vi "ParticleSwarmCore.vi"(4 "Stop notifier":refnum<notifier>, 5 "Fitness Function Data":variant, 6 "Parameters":T1={"Swarm size"=100, "Generations no."=500, "Cognitive coeff a1"=6.0, "Social coeff a2"=0.85, "Min inertia weight"=0.0, "Max inertia weight "=0.9, "Fmax"=0} {"Generations no." min=1; "Swarm size" min=1}, 7 "Fitness Function":T2, 8 "Population notifier":refnum<notifier>, 9 "Solution Progress notifier":refnum<notifier>, 10 "Satysfing fitness":dbl=inf, 11 "Phenotype size":i32) -> (0 "Generation":i32, 1 "fitness":dbl, 3 "Solution":i32[](array[numeric]))   [LabVIEW 2016, in "Optimal Frequency Bands Search.lvlib" / "ParticleSwarm.lvlib"]
doc: "Процедура, реализующая алгоритм роя частиц."
uses:
  ParticleSwarm.lvlib
  tFitness Function.ctl
  PSO_tParameters.ctl
  PSO_tPopulation.ctl
  PSO_tSolution progress.ctl
panel:
  # "This VI is a part of BCI Design library, http://www.ru-bci.org \nCopyright © 2020, Sotnikov Peter, All rights reserved. License: GNU GPLv3"
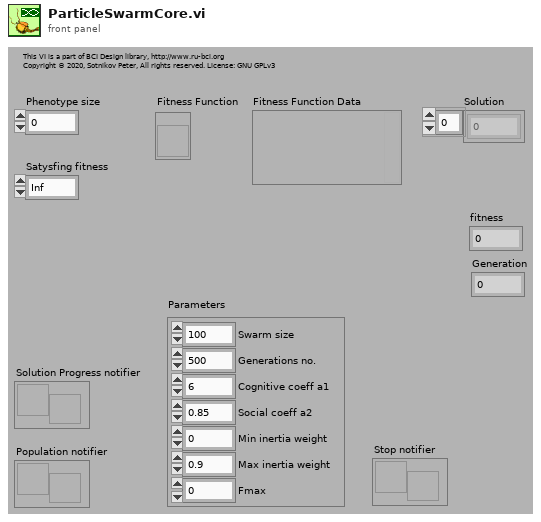
[diagram p1: front panel]
types:
  T1 = typedef "Optimal Frequency Bands Search.lvlib/ParticleSwarm.lvlib/PSO_tParameters.ctl" = cluster{"Swarm size":i32, "Generations no.":i32, "Cognitive coeff a1":dbl, "Social coeff a2":dbl, "Min inertia weight":dbl, "Max inertia weight ":dbl, "Fmax":i32}
  T2 = typedef "Optimal Frequency Bands Search.lvlib/ParticleSwarm.lvlib/tFitness Function.ctl" = refnum<vi>
  T3 = typedef "Optimal Frequency Bands Search.lvlib/ParticleSwarm.lvlib/PSO_tSolution progress.ctl" = cluster{"Solution":i32[], "Fitness":dbl, "Inertia":dbl, "Generation":i32}
  T4 = typedef "Optimal Frequency Bands Search.lvlib/ParticleSwarm.lvlib/PSO_tPopulation.ctl" = cluster{"Particle Coordinates":i32[][], "Fitnesses":dbl[], "Sorted indices":i32[], "Pbest Fitnesses":dbl[], "Pbest Particle Coordinates":i32[][], "Previous Velocity":dbl[][]}
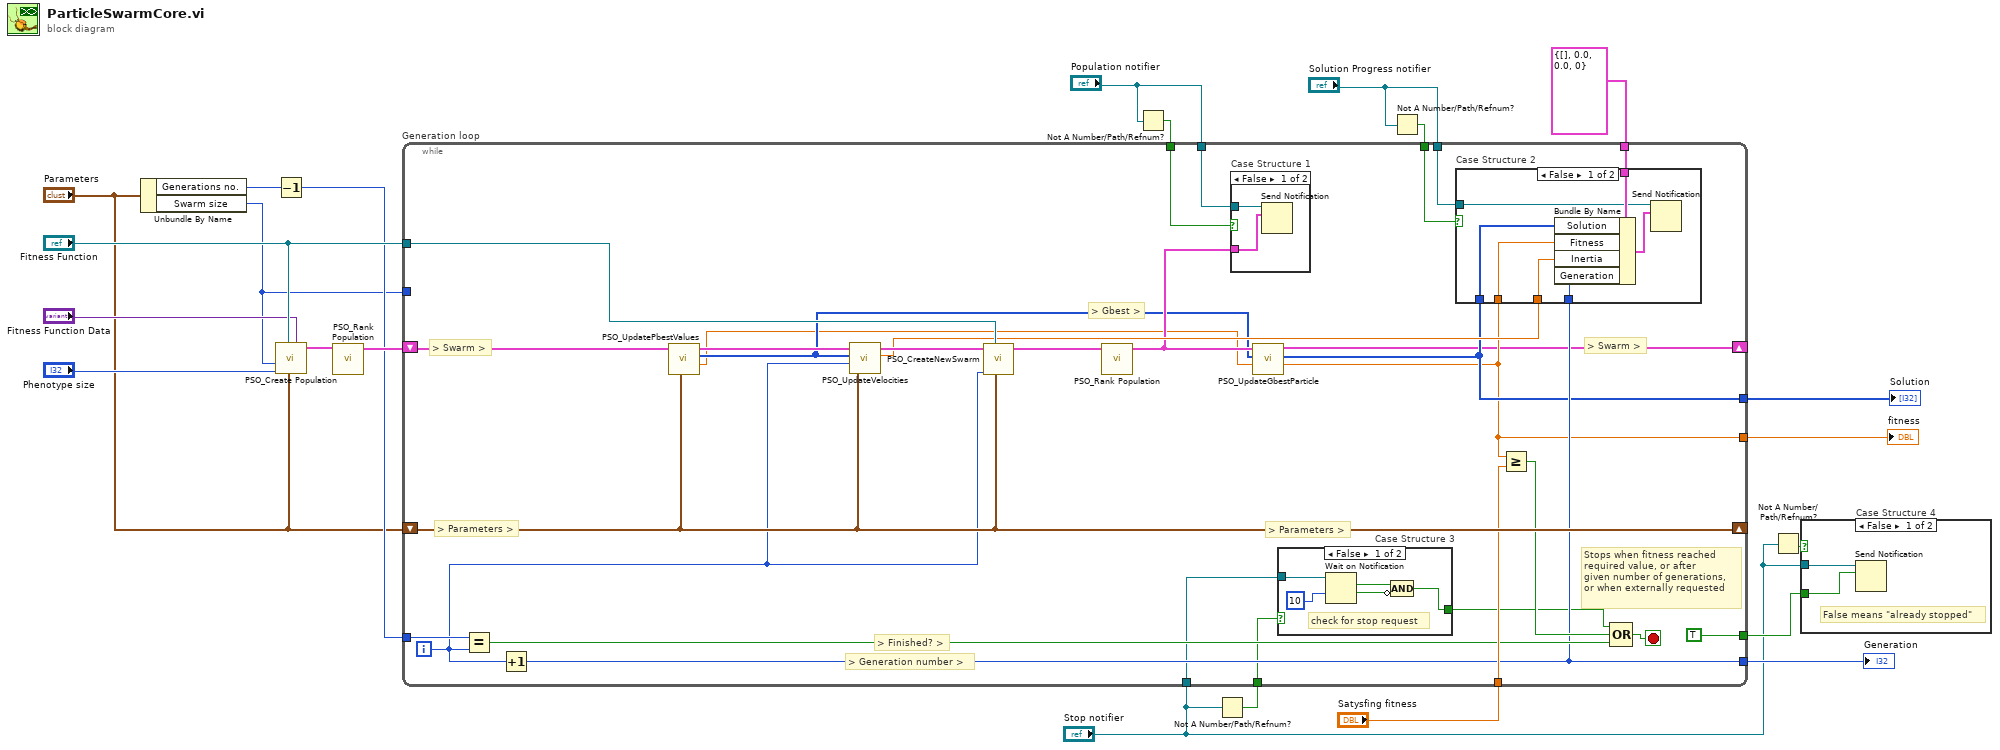
[diagram p0: block diagram]
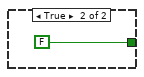
[diagram p3: hidden frame]
diagram:
  n1 = Unbundle By Name("Parameters") -> ("Generations no."=w17:i32, "Swarm size"=w4:i32)
  n2 = Decrement(x=w17) -> (x-1=w16:i32)
  n3 = call "PSO_Create Population.vi"("Function Data"="Fitness Function Data", "Parameters"="Parameters", "Fitness Function"="Fitness Function", "Phenotype size"="Phenotype size", "Population size"=w4) -> ("Population out"=w21:T4)  [unwired: 6 in]
  n4 = call "PSO_Rank Population.vi"("Population in"=w21) -> ("Population out"=w20:T4)  [unwired: 10 in]
  n5 = Not A Number/Path/Refnum?(number/path/refnum="Population notifier") -> (NaN/Path/Refnum?=w9:bool)
  n6 = Not A Number/Path/Refnum?(number/path/refnum="Stop notifier") -> (NaN/Path/Refnum?=w5:bool)
  n7 = Not A Number/Path/Refnum?(number/path/refnum="Solution Progress notifier") -> (NaN/Path/Refnum?=w7:bool)
  n8 = while "Generation loop" {
    tunnel: w4 -> [_]
    shift-right: [w24] -> _
    shift-left: w20 -> [w50]
    shift-right: [w51] -> _
    shift-left: "Parameters" -> [w51]
    tunnel: "Fitness Function" -> [w49]
    tunnel: w16 -> [w48]
    tunnel: "Satysfing fitness" -> [w47]
    tunnel: "Population notifier" -> [w38]
    tunnel: T3 {"Solution"=[], "Fitness"=0.0, "Inertia"=0.0, "Generation"=0} ("Solution progress") -> [w43]
    tunnel: [w42] -> w14
    tunnel: "Solution Progress notifier" -> [w37]
    tunnel: "Stop notifier" -> [w39]
    tunnel: [TRUE] -> w11
    tunnel: w9 -> [w36]
    tunnel: w7 -> [w35]
    tunnel: w5 -> [w34]
    tunnel: [w26] -> w3
    tunnel: [w25] -> w2
    i -> [w23]
    stop <- w46 stop-if-true
    # "> Gbest >"
    # "> Finished? >"
    # "> Generation number >"
    # "Stops when fitness reached\nrequired value, or after\ngiven number of generations,\nor when externally requested"
    # "> Parameters >"
    # "> Swarm >"
    # "> Parameters >"
    # "> Swarm >"
    n9 = Equal?(x=w48, y=w23) -> (x = y?=w45:bool)
    n10 = Increment(x=w23) -> (x+1=w42:i32)
    n11 = call "PSO_UpdatePbestValues.vi"("Parameters"=w51, "Population in"=w50) -> ("GBest Fitness"=w27:dbl, "Gbest Particle"=w28:i32[], "Population out"=w33:T4)  [unwired: 7 in]
    n12 = call "PSO_UpdateVelocities.vi"("Parameters in"=w51, "Generation"=w23, "Gbest Particle"=w28, "Population"=w33) -> ("Inertia Weight"=w30:dbl, "Population out"=w32:T4)  [unwired: 6 in]
    n13 = call "PSO_CreateNewSwarm.vi"("Parameters"=w51, "Fitness Function"=w49, "Generation"=w23, "Population in"=w32) -> ("Population out"=w31:T4)  [unwired: 7 in]
    n14 = call "PSO_Rank Population.vi"("Population in"=w31) -> ("Population out"=w29:T4)  [unwired: 10 in]
    n15 = case "Case Structure 1" shown="False" w36 {
      tunnel: w38 -> [w66 _]
      tunnel: w29 -> [w65 _]
      frame False {
        n16 = Send Notification(notification=w65, notifier=w66) -> ()  [unwired: 1 in, 2 out]
      }
      frame True {
      }
    }
    n17 = call "PSO_UpdateGbestParticle.vi"("Gbest Fitness"=w27, "Gbest Particle"=w28, "Population in"=w29) -> ("Fitness"=w25:dbl, "Solution"=w26:i32[], "Population out"=w24:T4)  [unwired: 6 in]
    n18 = case "Case Structure 3" shown="False" w34 {
      tunnel: [w52 FALSE ("ignore previous (T)")] -> w41
      tunnel: w39 -> [w56 _]
      frame False {
        # "check for stop request"
        n19 = Wait on Notification(notifier=w56, timeout in ms (-1)=10 ("ms timeout (-1)")) -> (notification=w53:bool, timed out?=w54:bool)  [unwired: 2 in, 2 out]
        n20 = Compound Arithmetic op=AND(w53, invert w54) -> (w52:bool)
      }
      frame True {
      }
    }
    n21 = case "Case Structure 2" shown="False" w35 {
      tunnel: w43 -> [w64 _]
      tunnel: w37 -> [w62 _]
      tunnel: w42 -> [w61 _]
      tunnel: w30 -> [w60 _]
      tunnel: w25 -> [w59 _]
      tunnel: w26 -> [w58 _]
      frame False {
        n22 = Bundle By Name(cluster=w64, "Solution"=w58, "Fitness"=w59, "Inertia"=w60, "Generation"=w61) -> (w63:T3)
        n23 = Send Notification(notification=w63, notifier=w62) -> ()  [unwired: 1 in, 2 out]
      }
      frame True {
      }
    }
    n24 = Greater Or Equal?(x=w25, y=w47) -> (x >= y?=w44:bool)
    n25 = Compound Arithmetic op=OR(w41, w44, w45) -> (w46:bool)
  }
  "Solution" <- w3
  "fitness" <- w2
  "Generation" <- w14
  n26 = Not A Number/Path/Refnum?(number/path/refnum="Stop notifier") -> (NaN/Path/Refnum?=w12:bool)
  n27 = case "Case Structure 4" shown="False" w12 {
    tunnel: "Stop notifier" -> [w68 _]
    tunnel: w11 -> [w67 _]
    frame False {
      # "False means \"already stopped\""
      n28 = Send Notification(notification=w67, notifier=w68) -> ()  [unwired: 1 in, 2 out]
    }
    frame True {
    }
  }
